vi "UTF-8 Conversion.vi"(7 "Unicode?":bool, 8 "error in":errorcluster, 11 "Config String":string) -> (0 "error out":errorcluster, 3 "Unicode/ANSI string":string)   [LabVIEW 2024]
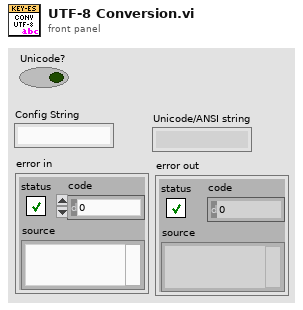
[diagram p1: front panel]
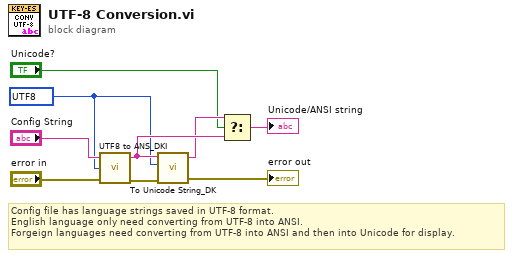
[diagram p0: block diagram]
diagram:
  w4 = 65001 items=["System default"=0, "Latin-1"=1252, "Japanese"=932, "Korean"=947, "Chinese simplified"=936, "Chinese traditional"=950, "Central Europe"=1250, "Cyrillic"=1251, "Greek"=1253, "Turkish"=1254, "Hebrew"=1255, "Arabic"=1256, "Baltic"=1257, "Thai"=874, "Vietnamese"=783, "UTF8"=65001, "UTF-7"=65000] ("Code Page")
  # "Config file has language strings saved in UTF-8 format.\nEnglish language only need converting from UTF-8 into ANSI.\nForgeign languages need converting from UTF-8 into ANSI and then into Unicode for display."
  n1 = call "UTF8 to ANS_DKI.vi"("error in"="error in", "Code Page"=w4, "UTF8 string"="Config String") -> ("error out"=w3:errorcluster, "ANSI/Multibyte string"=w9:string)  [unwired: 1 in]
  n2 = call "To Unicode String_DK.vi"("error in"=w3, "Code Page"=w4, "Multibyte String"=w9) -> ("error out"=→"error out":errorcluster, "Unicode string"=w8:string)  [unwired: 2 in]
  n3 = Select(t=w8, s="Unicode?", f=w9) -> (s? t:f=→"Unicode/ANSI string":string)
